vi "test_riccat_04Ni.vi"() -> (3 "All Tests Passed":bool)   [LabVIEW 2019]
uses:
  <vilib>/Analysis/Matrix/Datatypes/RealMatrix.ctl
  <vilib>/Analysis/7linalg.llb/Real Transpose Matrix.vi
  <vilib>/Analysis/7linalg.llb/Solve Linear Equations (multiple right hand).vi
  <vilib>/Rock Robotics/WPI/ThirdParty/JAS_Junk/TrajLib/Trajectory_Library.lvlib
  <vilib>/Analysis/NI_AALPro.lvlib
  <vilib>/Analysis/Matrix/NI_Matrix.lvlib
panel:
  out "error 2":i32
  out "error":i32
  out "Solution Matrix":T1
  out "ScrA":T1
  out "ScrQ":T1
  out "R1":T1
  out "Q1":T1
  out "N1":T1
  in  "N":T1=[[1.0, 0.0], [0.0, 1.0]]
  out "error out 2":errorcluster
  out "Pos Semi Definite":bool
  out "Q_Chk_Passed":bool
  out "C":T1
  out "Q Check":T1
  out "Bad":bool
  out "Stable Bad":bool
  out "error out":errorcluster
  out "Eigenvalues":cdb[](array[numeric])
  out "Error":bool
  out "Iterations":i32
  out "Elapsed \nTime MS":dbl
  out "ZERO":T1
  out "X  Answer":T1
  in  "R":T1=[[1.0, 0.0], [0.0, 1.0]]
  in  "Q":T1=[[1.0, 0.0], [0.0, 1.0]]
  in  "B":T1=[[1.0, 0.0], [0.0, 1.0]]
  in  "A":T1=[[1.0, 0.0], [0.0, 1.0]]
  # "// ------------------------------------------------------------\n  // Test 4: A = B = Q = R = I_2 (2-by-2 identity matrix)"
  # "A4 << \n           1, 0, \n            0, 1;"
  # "B4 << \n    1, \n    0, \n    0, \n    1;"
  # "Solution weight ??"
  # "Q4 << \n        1, 0, \n         0, 1;"
  # "Cost ??"
  # "R4 << \n        1, 0, \n        0, 1;"
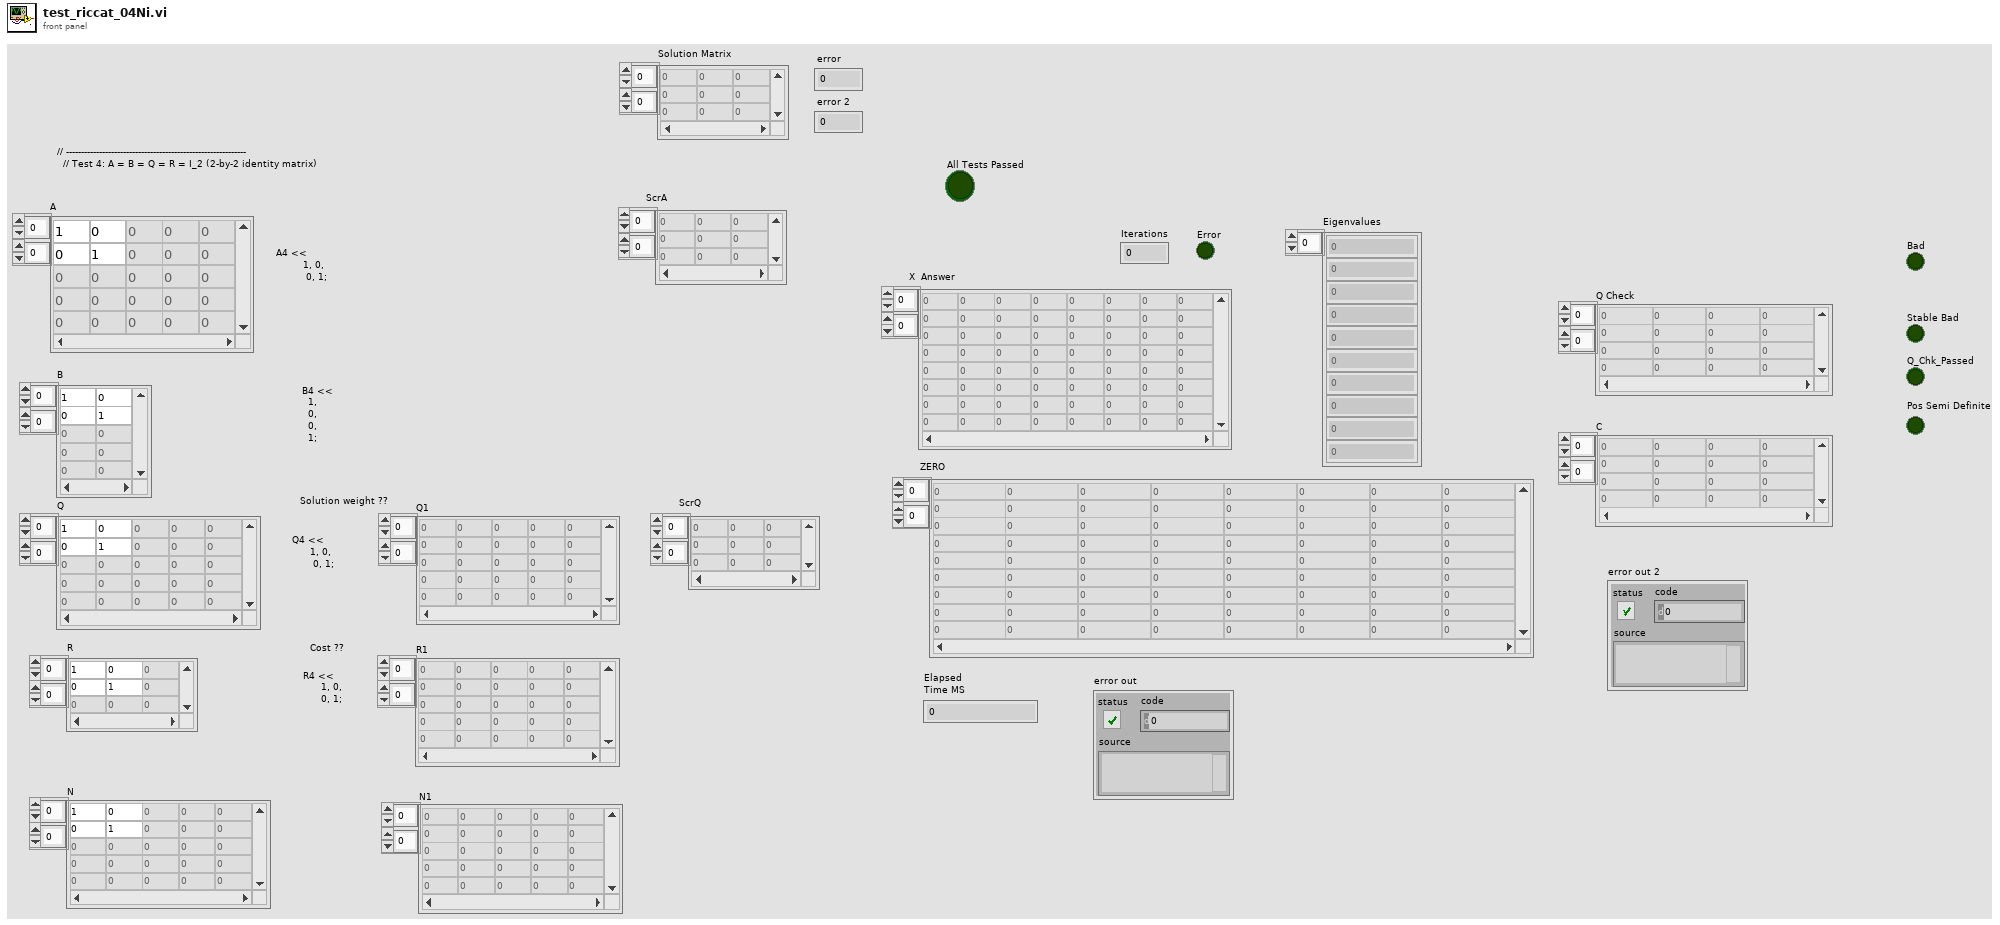
[diagram p1: front panel]
types:
  T1 = typedef "NI_Matrix.lvlib/RealMatrix.ctl" = dbl[][]
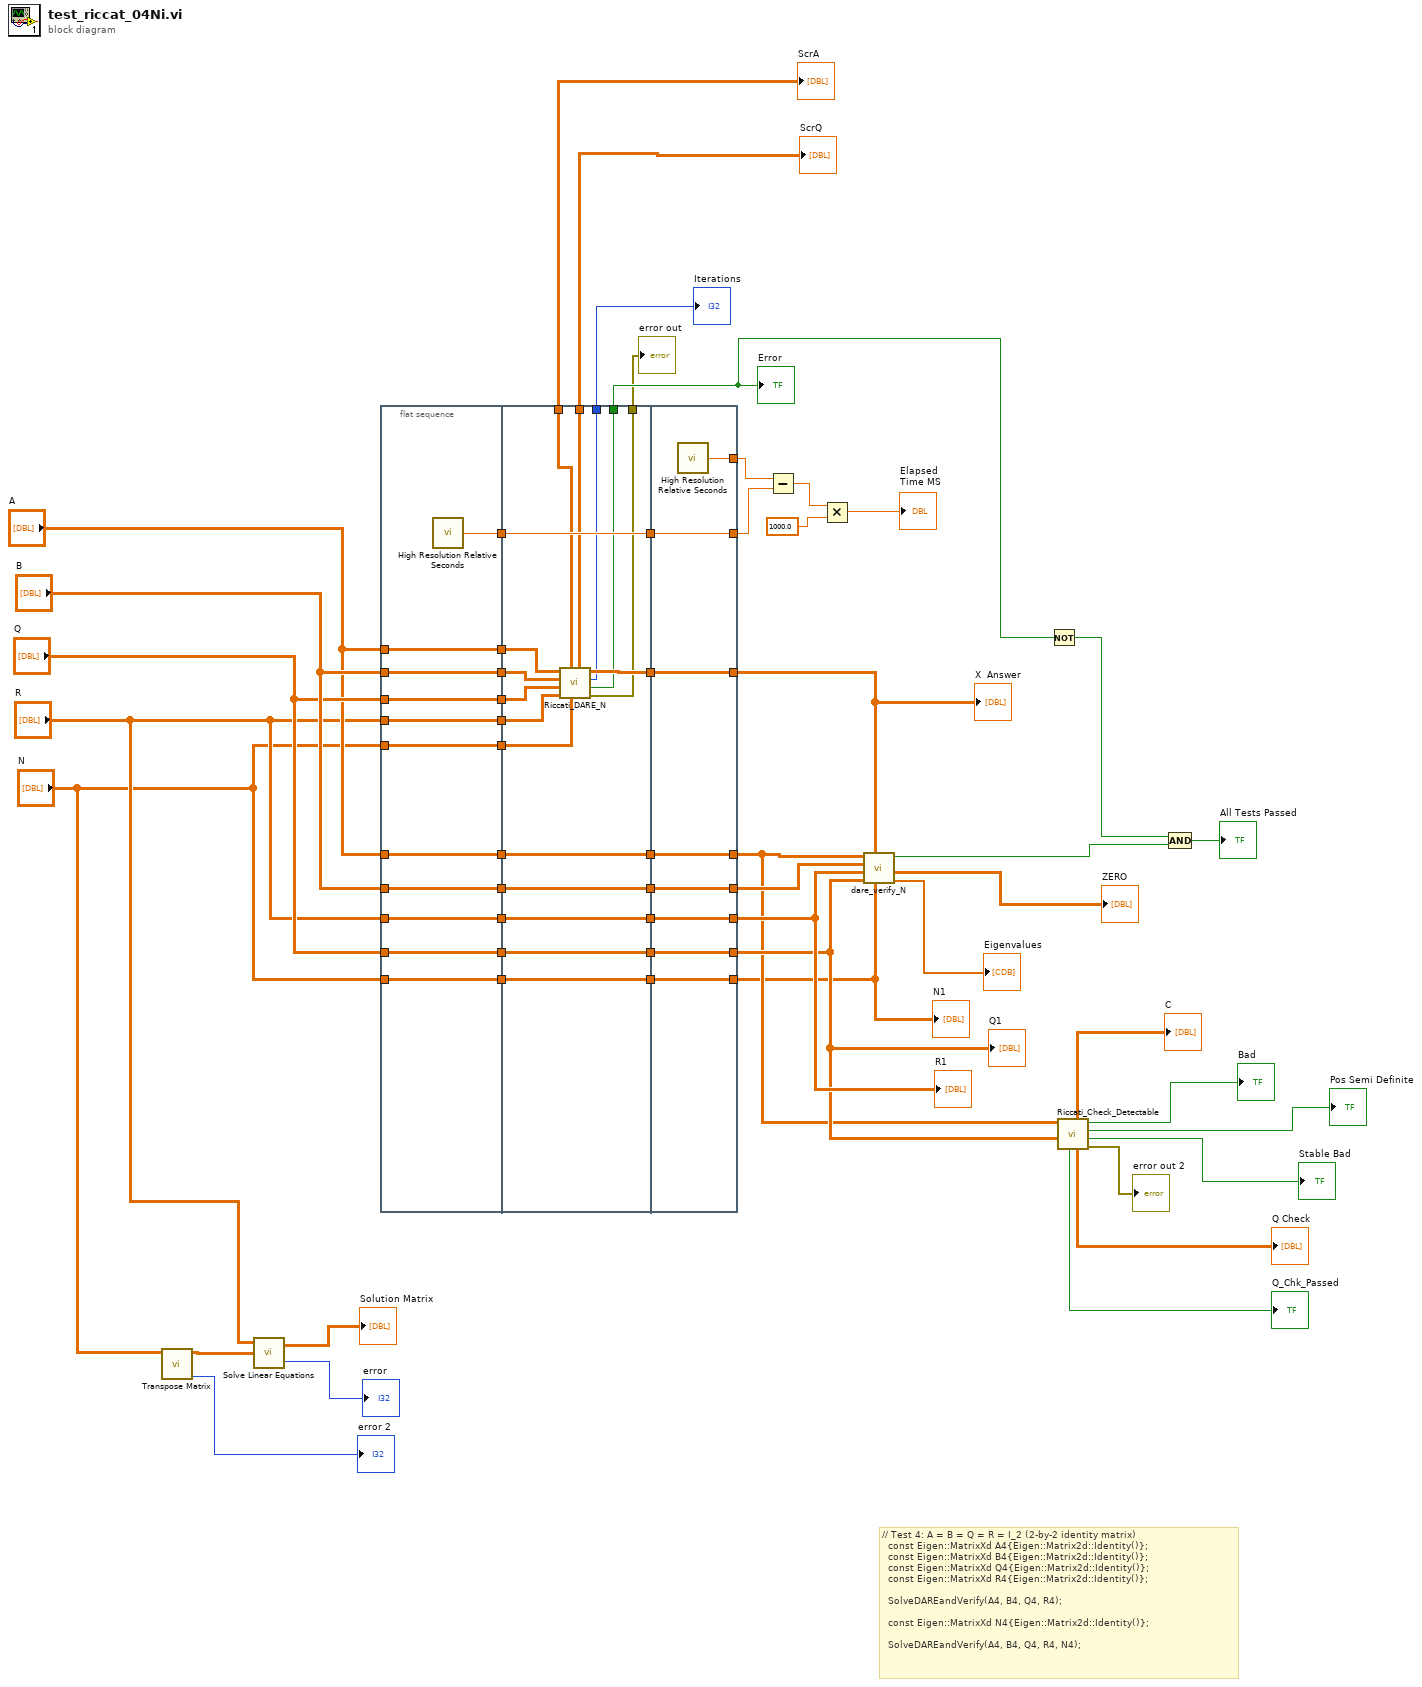
[diagram p0: block diagram]
diagram:
  # "// Test 4: A = B = Q = R = I_2 (2-by-2 identity matrix)\n  const Eigen::MatrixXd A4{Eigen::Matrix2d::Identity()};\n  const Eigen::MatrixXd B4{Eigen::Matrix2d::Identity()};\n  const Eigen::MatrixXd Q4{Eigen::Matrix2d::Identity()};\n  const Eigen::MatrixXd R4{Eigen::Matrix2d::Identity()};\n\n  SolveDAREandVerify(A4, B4, Q4, R4);\n\n  const Eigen::MatrixXd N4{Eigen::Matrix2d::Identity()};\n\n  SolveDAREandVerify(A4, B4, Q4, R4, N4);"
  n1 = call-poly <vilib>:"Transpose Matrix.vi"("Input Matrix"="N") -> ("error"=→"error 2":i32, "Matrix Transpose"=w5:T1)  [unwired: 9 in]
  n2 = call-poly <vilib>:"Solve Linear Equations.vi"("Known Matrix"=w5, "Input Matrix"="R") -> ("error"=→"error":i32, "Solution Matrix"=→"Solution Matrix":T1)  [unwired: 1 in]
  n3 = flat-sequence {
    tunnel: "B" -> [w61]
    tunnel: "A" -> [w62]
    tunnel: "B" -> [w63]
    tunnel: "Q" -> [w64]
    tunnel: "A" -> [w65]
    tunnel: "R" -> [w66]
    tunnel: [w66] -> w55
    tunnel: [w65] -> w54
    tunnel: [w64] -> w53
    tunnel: [w63] -> w52
    tunnel: [w62] -> w51
    tunnel: [w61] -> w50
    tunnel: "R" -> [w60]
    tunnel: [w60] -> w45
    tunnel: "Q" -> [w59]
    tunnel: [w59] -> w44
    tunnel: [w58] -> w39
    tunnel: [w57] -> w14
    tunnel: "N" -> [w57]
    tunnel: "N" -> [w56]
    tunnel: [w56] -> w11
    tunnel: w55 -> [w83]
    tunnel: w54 -> [w81]
    tunnel: w53 -> [w80]
    tunnel: w52 -> [w79]
    tunnel: w51 -> [w78]
    tunnel: w50 -> [w77]
    tunnel: [w82] -> w49
    tunnel: [w78] -> w48
    tunnel: [w77] -> w47
    tunnel: [w76] -> w46
    tunnel: w45 -> [w76]
    tunnel: w44 -> [w75]
    tunnel: [w75] -> w43
    tunnel: [w74] -> w40
    tunnel: w39 -> [w74]
    tunnel: [w73] -> w35
    tunnel: [w72] -> w34
    tunnel: [w71] -> w26
    tunnel: w14 -> [w70]
    tunnel: [w69] -> w12
    tunnel: w11 -> [w69]
    tunnel: [w68] -> w8
    tunnel: [w67] -> w7
    tunnel: [w89] -> w22
    tunnel: [w90] -> w20
    tunnel: [w91] -> w33
    tunnel: w49 -> [w91]
    tunnel: w48 -> [w90]
    tunnel: w47 -> [w89]
    tunnel: [w88] -> w32
    tunnel: w46 -> [w88]
    tunnel: w43 -> [w85]
    tunnel: [w87] -> w42
    tunnel: [w86] -> w41
    tunnel: w40 -> [w86]
    tunnel: [w85] -> w21
    tunnel: [w84] -> w13
    tunnel: w12 -> [w84]
    frame #0 {
      n4 = call <vilib>:"High Resolution Relative Seconds.vi"() -> ("relative seconds"=w58:dbl)
    }
    frame #1 {
      n5 = call <vilib>:"Riccati_DARE_N.vi"("N"=w70, "R"=w83, "Q"=w80, "B"=w79, "A"=w81) -> ("error out"=w71:errorcluster, "Error"=w72:bool, "Iterations"=w73:i32, "Answer"=w82:T1, "ScrQ"=w68:T1, "ScrA"=w67:T1)  [unwired: 1 in]
    }
    frame #2 {
      n6 = call <vilib>:"High Resolution Relative Seconds.vi"() -> ("relative seconds"=w87:dbl)
    }
  }
  n7 = Subtract(x=w42, y=w41) -> (x-y=w38:dbl)
  n8 = Multiply(x=w38, y=1000.0) -> (x*y=→"Elapsed \nTime MS":dbl)
  n9 = call "dare_verify_N.vi"("N"=w13, "Answer"=w33, "Q"=w21, "R"=w32, "B"=w22, "A"=w20) -> ("Eigenvalues"=→"Eigenvalues":cdb[], "ZERO"=→"ZERO":T1, "Passed"=w29:bool)  [unwired: 3 in]
  n10 = Not(x=w34) -> (.not. x?=w30:bool)
  n11 = call <vilib>:"Riccati_Check_Detectable.vi"("Q"=w21, "A"=w20) -> ("error out"=→"error out 2":errorcluster, "Stable Bad"=→"Stable Bad":bool, "Pos Semi Definite"=→"Pos Semi Definite":bool, "Bad"=→"Bad":bool, "Q_Check"=→"Q Check":T1, "C"=→"C":T1, "Q_Chk_Passed"=→"Q_Chk_Passed":bool)  [unwired: 3 in]
  n12 = Compound Arithmetic op=AND(w30, w29) -> (→"All Tests Passed":bool)
  "X  Answer" <- w33
  "Iterations" <- w35
  "Error" <- w34
  "error out" <- w26
  "N1" <- w13
  "Q1" <- w21
  "R1" <- w32
  "ScrQ" <- w8
  "ScrA" <- w7
